vi "项操作.vi"(8 "error in (no error)":errorcluster caption="错误输入（无错误）", 9 "Cell Position":T1, 10 "MCListbox引用句柄":refnum<vi>, 11 "LNK 输入":refnum<class "UP.lvclass">) -> (0 "error out":errorcluster caption="错误输出", 3 "LNK 输出":refnum<class "UP.lvclass">)   [LabVIEW 2016, in "UP.lvclass"]
uses:
  UP.lvclass
  <vilib>/Utility/miscctls.llb/LVRowAndColumnTypeDef.ctl
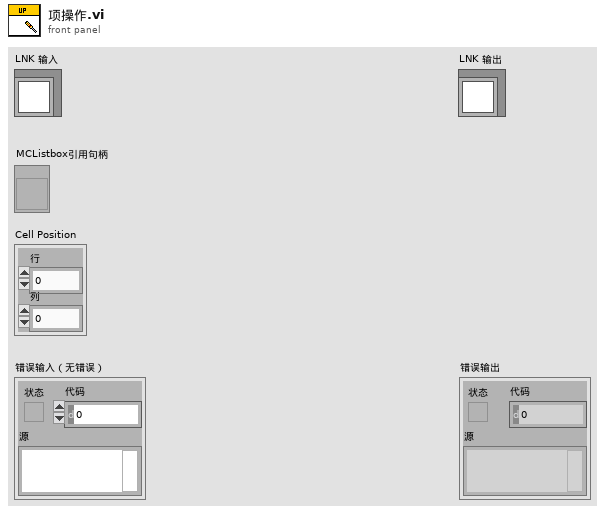
[diagram p1: front panel]
types:
  T1 = typedef "LVRowAndColumnTypeDef.ctl" = cluster{"Row":i32, "Column":i32}
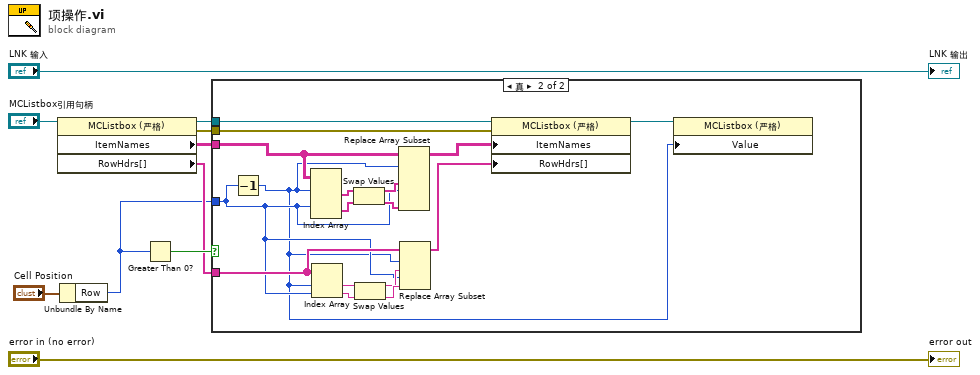
[diagram p0: block diagram]
diagram:
  n1 = property class="MCListbox (严格)"(reference="MCListbox引用句柄") -> (reference out=w7:refnum<vi>, error out=w6:errorcluster, "ItemNames"=w4:string[][], "RowHdrs[]"=w3:string[])  [unwired: 1 in]
  n2 = Unbundle By Name("Cell Position") -> ("Row"=w1:i32)
  n3 = Greater Than 0?(x=w1) -> (x > 0?=w5:bool)
  n4 = case shown="真" w5 {
    tunnel: w7 -> [_ w27]
    tunnel: w6 -> [_ w26]
    tunnel: w4 -> [_ w25]
    tunnel: w1 -> [_ w12]
    tunnel: w3 -> [_ w13]
    frame False {
    }
    frame True {
      n5 = Decrement(x=w12) -> (x-1=w11:i32)
      n6 = Index Array(array=w25, index (row) #1=w11, index (row) #2=w12) -> (element #1=w22:string[], element #2=w20:string[])  [unwired: 2 in]
      n7 = Index Array(array=w13, index #1=w11, index #2=w12) -> (element #1=w15:string, element #2=w17:string)
      n8 = Swap Values(12:w22, 14:w20) -> (1:w21:string[], 3:w19:string[])  [unwired: 1 in]
      n9 = Swap Values(12:w15, 14:w17) -> (1:w16:string, 3:w18:string)  [unwired: 1 in]
      n10 = Replace Array Subset(array=w25, new element #1=w21, index (row) #1=w11, new element #2=w19, index (row) #2=w12) -> (w24:string[][])  [unwired: 2 in]
      n11 = Replace Array Subset(array=w13, new element #1=w16, index #1=w11, new element #2=w18, index #2=w12) -> (w14:string[])
      n12 = property class="MCListbox (严格)"(reference=w27, error in=w26, "ItemNames"=w24, "RowHdrs[]"=w14) -> (reference out=w23:refnum<vi>)  [unwired: 1 out]
      n13 = property class="MCListbox (严格)"(reference=w23, "Value"=w11) -> ()  [unwired: 1 in, 2 out]
    }
  }
  "error out" <- "error in (no error)"
  "LNK 输出" <- "LNK 输入"
